vi "psum and nsum.vi"() -> ()   [LabVIEW 2013]
panel:
  out "nsum":dbl
  out "psum":dbl
  in  "Array 3":dbl[](array[numeric])
  out "Array 2":string[](array[string])
  in  "Array":dbl[](array[numeric])
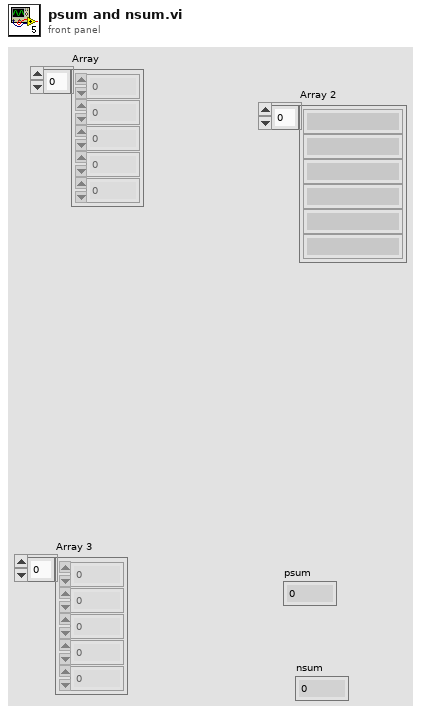
[diagram p1: front panel]
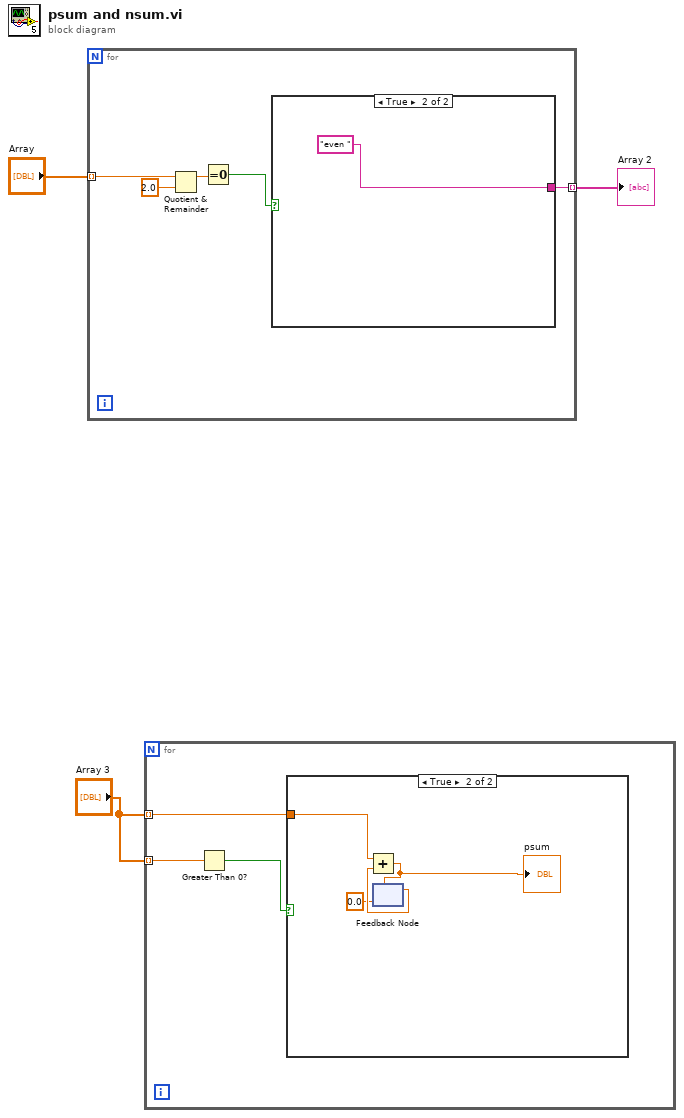
[diagram p0: block diagram]
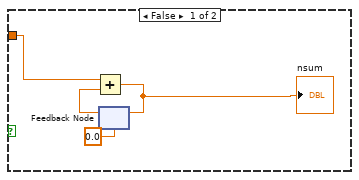
[diagram p2: hidden frame]
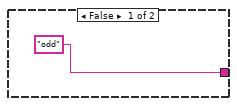
[diagram p3: hidden frame]
diagram:
  n1 = for {
    tunnel: "Array" -> [w8] mode=indexing
    tunnel: [w4] -> w2 mode=indexing
    n2 = Quotient & Remainder(x=w8, y=2.0) -> (x-y*floor(x/y)=w6:dbl)  [unwired: 1 out]
    n3 = Equal To 0?(x=w6) -> (x = 0?=w7:bool)
    n4 = case shown="True" w7 {
      tunnel: ["odd" "even "] -> w4
      frame False {
      }
      frame True {
      }
    }
  }
  "Array 2" <- w2
  n5 = for {
    tunnel: "Array 3" -> [w13] mode=indexing
    tunnel: "Array 3" -> [w11] mode=indexing
    n6 = Greater Than 0?(x=w13) -> (x > 0?=w12:bool)
    n7 = case shown="True" w12 {
      tunnel: w11 -> [w17 w21]
      frame False {
        n8 = feedback #1(0.0) -> (w16:dbl)
        n9 = Add(x=w17, y=w16) -> (x+y=w14:dbl)
        "nsum" <- w14
        n10 = feedback-in #1(w14) -> ()
      }
      frame True {
        n11 = feedback #2(0.0) -> (w20:dbl)
        n12 = Add(x=w21, y=w20) -> (x+y=w18:dbl)
        "psum" <- w18
        n13 = feedback-in #2(w18) -> ()
      }
    }
  }
